vi "PolarToCartesian.vi"(10 "theta (radians)":dbl, 11 "r":dbl) -> (2 "y":dbl, 3 "x":dbl)   [LabVIEW 2013]
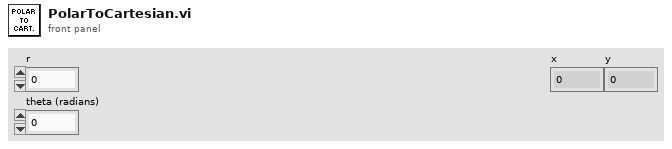
[diagram p1: front panel]
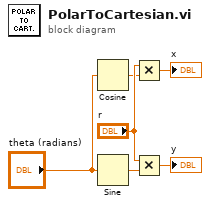
[diagram p0: block diagram]
diagram:
  n1 = Cosine(x="theta (radians)") -> (cos(x)=w3:dbl)
  n2 = Sine(x="theta (radians)") -> (sin(x)=w4:dbl)
  n3 = Multiply(x="r", y=w3) -> (x*y=→"x":dbl)
  n4 = Multiply(x="r", y=w4) -> (x*y=→"y":dbl)
